vi "Insertar_Objeto_Base.vi"(4 "Error":dbl, 6 "Base":T1, 7 "Puntos Fotos":T1, 8 "Dimensión k del espacio":u8, 9 "Vector promedio c":dbl[](array[numeric]), 10 "# Fotos":i32, 11 "Nombre del objeto":string) -> ()   [LabVIEW 2020]
doc: "Este VI recibe el nombre del objeto, una matriz que contiene la base del objeto, las coordenadas en el espacio generado por la base de cada imagen tomada a diferentes rotaciones del objeto, el vector promedio de las imágenes, el número de puntos, la dimensión k del espacio y el error. Cada uno de estos parámetros son mandados a la base de datos específicada por el archivo .udl de la variable global Path."
uses:
  <vilib>/Analysis/Matrix/Datatypes/RealMatrix.ctl
  <vilib>/addons/database/Auxilliary.llb/DB Tools Parameter Info.ctl
  <vilib>/addons/database/Auxilliary.llb/DB Tools DataTypes.ctl
  <vilib>/addons/database/Auxilliary.llb/DB Tools Parameter Dir.ctl
  <vilib>/Analysis/Matrix/Numeric/Conversions/Matrix To Array - RM.vi
  Global_archivobasedatos.vi
  <vilib>/addons/database/Connection.llb/DB Tools Open Connec (Path).vi
  <vilib>/addons/database/Command.llb/Cmd Set Parameter Value (C).vi
  <vilib>/addons/database/Command.llb/Cmd Execute.vi
  <vilib>/addons/database/Recordset.llb/Rec Destroy - Command.vi
  <vilib>/addons/database/Command.llb/Cmd Get String Parameter Value (C).vi
  <vilib>/addons/database/Command.llb/Cmd Delete.vi
  <vilib>/addons/database/NI_Database_API.lvlib
  <vilib>/Analysis/Matrix/NI_Matrix.lvlib
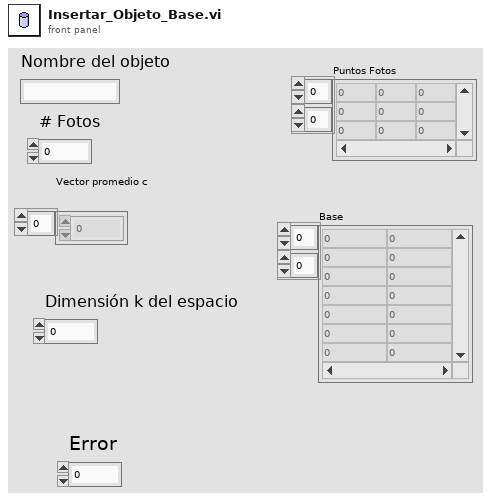
[diagram p1: front panel]
types:
  T1 = typedef "NI_Matrix.lvlib/RealMatrix.ctl" = dbl[][]
  T2 = typedef "NI_Database_API.lvlib/DB Tools Parameter Info.ctl" = cluster{"parameter name":string, "type":T3, "direction":T4, "value":variant}
  T3 = typedef "NI_Database_API.lvlib/DB Tools DataTypes.ctl" = enum16{"String", "Long (I32)", "Single (SGL)", "Double (DBL)", "Date/Time", "Binary"}
  T4 = typedef "NI_Database_API.lvlib/DB Tools Parameter Dir.ctl" = enum32{"Input", "Output", "Input/Output", "Return Value"}
  T5 = typedef "NI_Database_API.lvlib/Conn ObjectReference.ctl" = refnum<k1>
  T6 = typedef "NI_Database_API.lvlib/Cmd ObjectReference.ctl" = refnum<k1>
  T7 = typedef "NI_Database_API.lvlib/Cmd-Rec Object Reference.ctl" = refnum<k1>
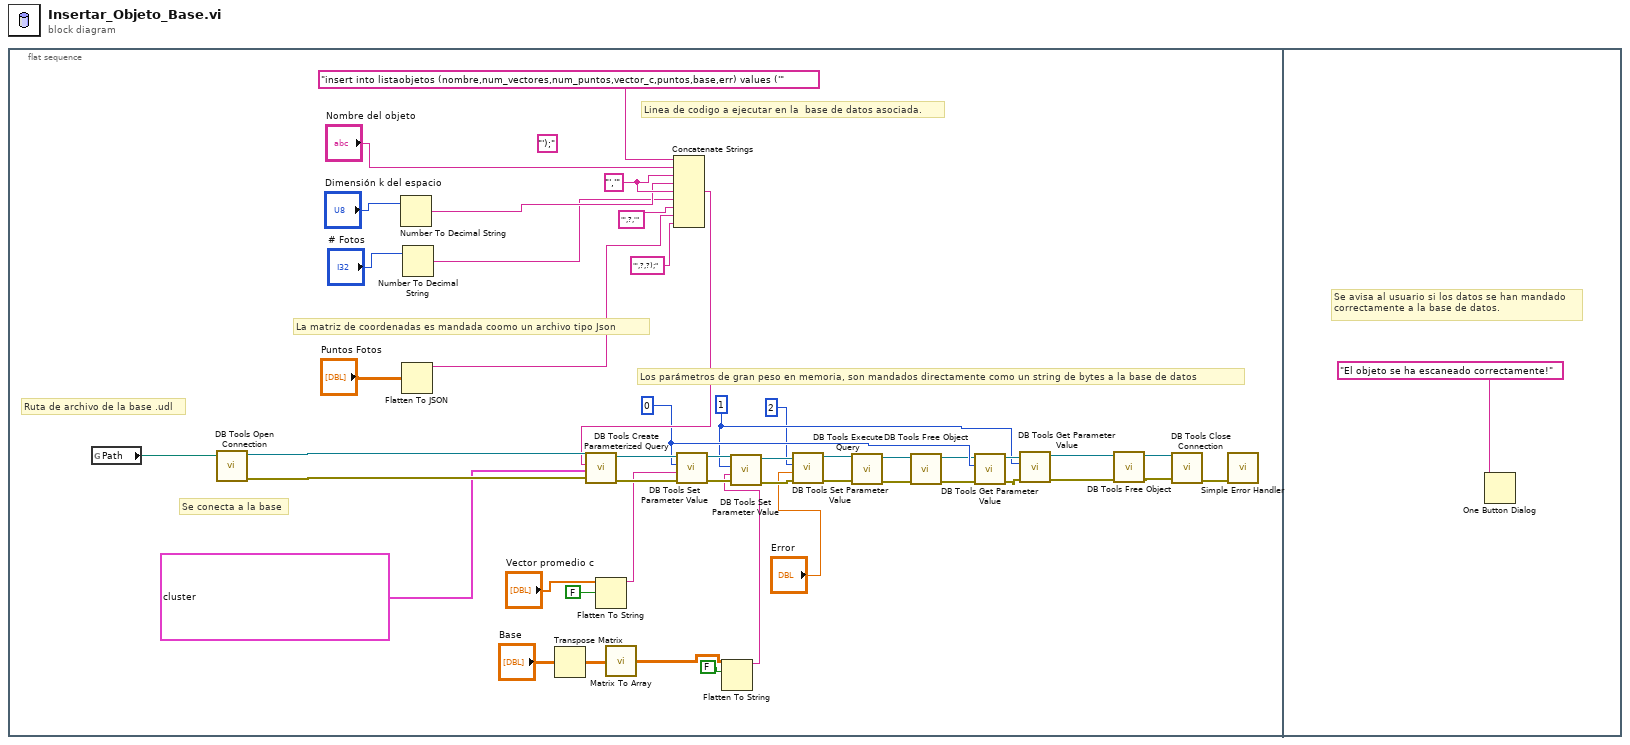
[diagram p0: block diagram]
diagram:
  n1 = flat-sequence {
    frame #0 {
      w11 = 1
      w23 = 0
      (unwired) "');" ("string")
      w42 = "','" ("string")
      # "La matriz de coordenadas es mandada coomo un archivo tipo Json"
      # "Los parámetros de gran peso en memoria, son mandados directamente como un string de bytes a la base de datos"
      # "Linea de codigo a ejecutar en la  base de datos asociada."
      # "Se conecta a la base"
      # "Ruta de archivo de la base .udl"
      n2 = global read "Global_archivobasedatos.vi" "Path"() -> (w47:path)
      n3 = call-poly <vilib>:"DB Tools Open Connection.vi"("connection information"=w47) -> ("error out"=w45:errorcluster, "connection reference"=w46:T5)  [unwired: 7 in]
      n4 = Number To Decimal String(number="Dimensión k del espacio") -> (decimal integer string=w36:string)  [unwired: 1 in]
      n5 = Flatten To JSON(anything="Puntos Fotos") -> (JSON string=w32:string)  [unwired: 2 in, 1 out]
      n6 = Number To Decimal String(number="# Fotos") -> (decimal integer string=w34:string)  [unwired: 1 in]
      n7 = Transpose Matrix(1:"Base") -> (0:w20:T1)
      n8 = Flatten To String(anything="Vector promedio c", prepend array or string size? (T)=FALSE) -> (data string=w26:string)  [unwired: 2 in, 2 out]
      n9 = call-poly <vilib>:"Matrix To Array.vi"("Real Matrix"=w20) -> ("Real 2D Array"=w17:dbl[][])
      n10 = Concatenate Strings("insert into listaobjetos (nombre,num_vectores,num_puntos,vector_c,puntos,base,err) values ('", "Nombre del objeto", w42, w36, w42, w34, "',?,'" ("string"), w32, "',?,?);" ("string")) -> (w30:string)
      n11 = call <vilib>:"DB Tools Create Parameterized Query.vi"("error in (no error)"=w45, "parameters"=T2[] [{"parameter name"="vectorc", "type"=enum."Binary", "direction"=enum."Input/Output", "value"=variant}, {"parameter name"="base", "type"=enum."Binary", "direction"=enum."Input/Output", "value"=variant}, {"parameter name"="err", "type"=enum."Double (DBL)", "direction"=enum."Input/Output", "value"=variant}], "SQL query"=w30, "connection reference"=w46) -> ("error out"=w27:errorcluster, "command reference"=w29:T6)  [unwired: 3 in, 1 out]
      n12 = call-poly <vilib>:"DB Tools Set Parameter Value.vi"("error in (no error)"=w27, "value"=w26, "parameter index"=w23, "command reference"=w29) -> ("error out"=w15:errorcluster, "command reference out"=w16:T6)  [unwired: 4 in]
      n13 = Flatten To String(anything=w17, prepend array or string size? (T)=FALSE) -> (data string=w14:string)  [unwired: 2 in, 2 out]
      n14 = call-poly <vilib>:"DB Tools Set Parameter Value.vi"("error in (no error)"=w15, "value"=w14, "parameter index"=w11, "command reference"=w16) -> ("error out"=w6:errorcluster, "command reference out"=w8:T6)  [unwired: 4 in]
      n15 = call-poly <vilib>:"DB Tools Set Parameter Value.vi"("error in (no error)"=w6, "value"="Error", "parameter index"=2, "command reference"=w8) -> ("error out"=w9:errorcluster, "command reference out"=w7:T6)  [unwired: 4 in]
      n16 = call-poly <vilib>:"DB Tools Execute Query.vi"("error in (no error)"=w9, "command reference"=w7) -> ("error out"=w41:errorcluster, "command-recordset reference"=w25:T7)  [unwired: 6 in]
      n17 = call-poly <vilib>:"DB Tools Free Object.vi"("error in (no error)"=w41, "command-recordset reference"=w25) -> ("error out"=w24:errorcluster, "command reference"=w22:T6)  [unwired: 8 in]
      n18 = call-poly <vilib>:"DB Tools Get Parameter Value.vi"("error in (no error)"=w24, "parameter index"=w23, "command reference"=w22) -> ("error out"=w12:errorcluster, "command reference out"=w13:T6)  [unwired: 4 in, 1 out]
      n19 = call-poly <vilib>:"DB Tools Get Parameter Value.vi"("error in (no error)"=w12, "parameter index"=w11, "command reference"=w13) -> ("error out"=w2:errorcluster, "command reference out"=w3:T6)  [unwired: 4 in, 1 out]
      n20 = call-poly <vilib>:"DB Tools Free Object.vi"("error in (no error)"=w2, "command reference"=w3) -> ("error out"=w10:errorcluster, "connection reference"=w4:T5)  [unwired: 8 in]
      n21 = call <vilib>:"DB Tools Close Connection.vi"("error in (no error)"=w10, "connection reference"=w4) -> ("error out"=w44:errorcluster)  [unwired: 5 in]
      n22 = call <vilib>:"Simple Error Handler.vi"("error in (no error)"=w44) -> ()  [unwired: 4 in, 5 out]
    }
    frame #1 {
      # "Se avisa al usuario si los datos se han mandado\ncorrectamente a la base de datos."
      n23 = One Button Dialog(message="El objeto se ha escaneado correctamente!") -> ()  [unwired: 1 in, 1 out]
    }
  }
